vi "q5 sum between p q for loop.vi"() -> ()   [LabVIEW 2025]
panel:
  out "SUM":dbl
  in  "Q":dbl
  in  "P":dbl
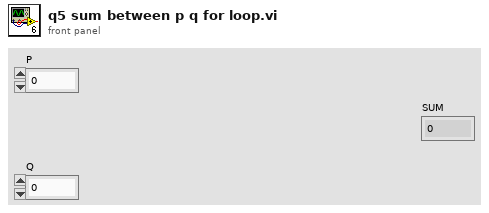
[diagram p1: front panel]
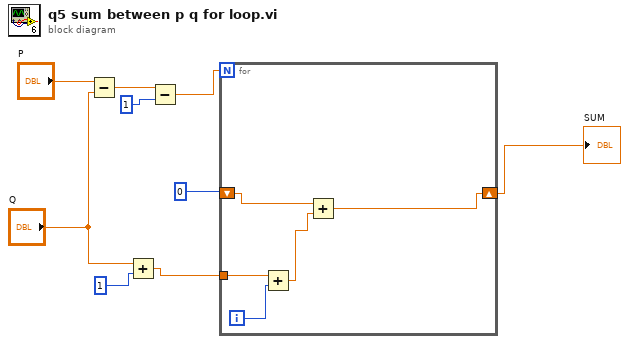
[diagram p0: block diagram]
diagram:
  n1 = Subtract(x="P", y="Q") -> (x-y=w8:dbl)
  n2 = Add(x="Q", y=1) -> (x+y=w2:dbl)
  n3 = Subtract(x=w8, y=1) -> (x-y=w6:dbl)
  n4 = for {
    N: w6 -> [_]
    shift-right: [w10] -> w1
    shift-left: 0 -> [w12]
    tunnel: w2 -> [w14]
    i -> [w13]
    n5 = Add(x=w14, y=w13) -> (x+y=w11:dbl)
    n6 = Add(x=w12, y=w11) -> (x+y=w10:dbl)
  }
  "SUM" <- w1
